vi "onDisconnection.vi"(8 "error in (no error)":errorcluster, 11 "TCPConnection in":refnum<class "TCPConnection.lvclass">) -> (0 "error out":errorcluster, 3 "No Connection":refnum<class "TCPConnection.lvclass">)   [LabVIEW 2013, in "MQTT_TCP.lvlib" / "TCPConnection.lvclass"]
uses:
  TCPConnection.lvclass
  MQTT_Connection/Connection/Connection.lvclass
  TCPConnection.lvclass/TCPConnection.ctl
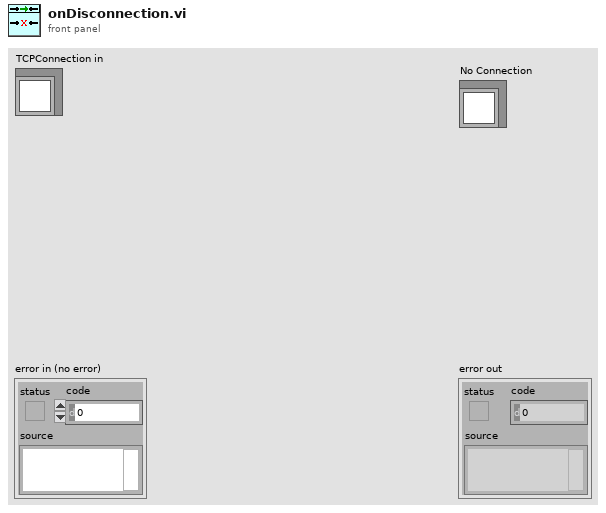
[diagram p1: front panel]
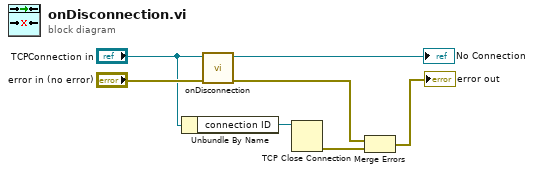
[diagram p0: block diagram]
diagram:
  n1 = Unbundle By Name("TCPConnection in") -> ("connection ID"=w5:refnum<k5>)
  n2 = call-parent "onDisconnection.vi"("error in (no error)"="error in (no error)", "Connection"="TCPConnection in") -> ("error out"=w3:errorcluster, "No connection"=→"No Connection":refnum<class "TCPConnection.lvclass">)  [unwired: 8 in]
  n3 = TCP Close Connection(connection ID=w5) -> (error out=w4:errorcluster)  [unwired: 2 in, 1 out]
  n4 = Merge Errors(w3, w4) -> (→"error out":errorcluster)
